vi "4155C Transfer Config SMUs.vi"(0 "VISA resource name in":refnum<visa-resource-name>, 1 "sweep method":u16(ring) items=["Continuous", "Pulsed"], 2 "Gate mode":u16(ring) items=["Auto", "Limited", "Fixed"], 3 "Gate Range":u8(slide)=6 max=11 scale=0.0..11.0, 5 "Pulse period":dbl=0.005 min=0.005 max=1.0 step=0.0001 format="%.4f", 7 "Pulse width":dbl=0.0005 min=0.0005 max=0.1 step=0.0001 format="%.4f", 8 "Drain Standby":bool, 9 "Base voltage":dbl format="%^.4e", 10 "Gate Standby":bool, 11 "error in (no error)":errorcluster, 12 "SMU4":cluster{"on/off":bool, "Voltage":dbl} {"Voltage" min=-100.0 max=100.0 format="%.2f"}, 13 "Source/drain mode":u16(ring) items=["Auto", "Limited", "Fixed"], 14 "Source/drain Range":u8(slide)=6 max=11 scale=0.0..11.0) -> (4 "VISA Resource Name out":refnum<visa-resource-name>, 15 "error out":errorcluster)   [LabVIEW 2016]
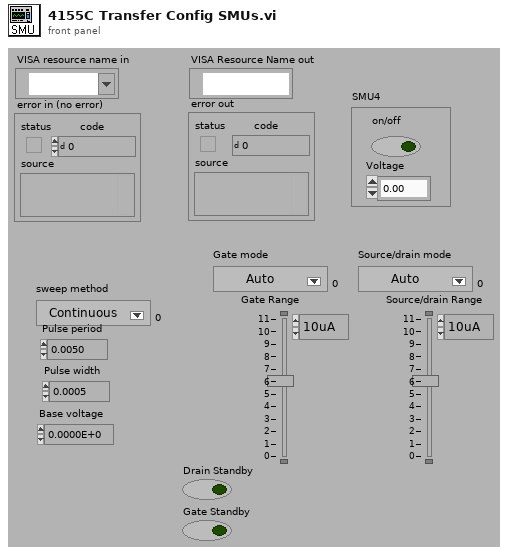
[diagram p1: front panel]
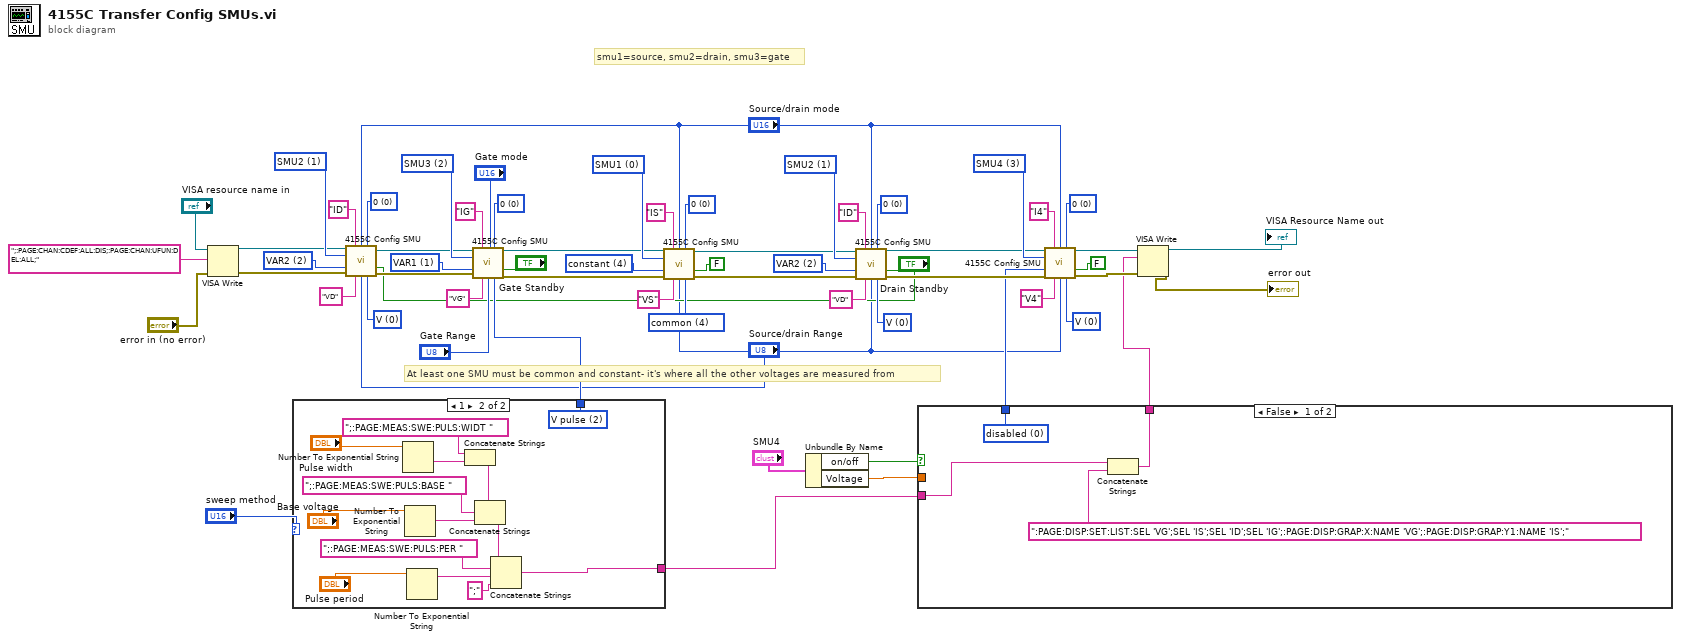
[diagram p0: block diagram]
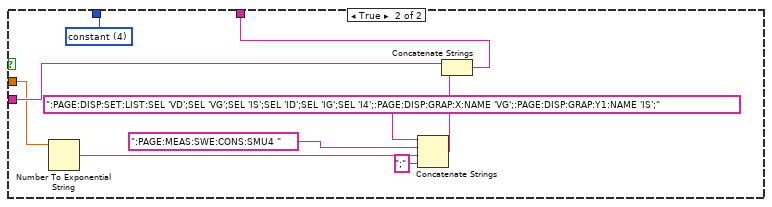
[diagram p2: hidden frame]
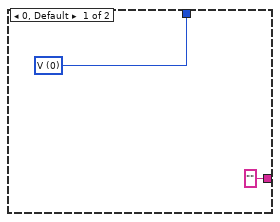
[diagram p3: hidden frame]
diagram:
  w18 = u32 1 items=["SMU1  ", "SMU2  ", "SMU3  ", "SMU4  ", "SMU5  ", "SMU6  "] ("unit to configure")
  w19 = u32 2 items=["disabled  ", "VAR1  ", "VAR2  ", "VAR1'  ", "constant  "] ("function")
  w21 = u32 0 items=["0  ", "10K Ohms  ", "100K Ohms  ", "1M Ohms  "] ("series resistance *")
  w22 = u32 0 items=["V  ", "I  ", "V pulse  ", "I pulse  ", "  common  "] ("mode")
  w40 = u32 0 items=["V  ", "I  ", "V pulse  ", "I pulse  ", "  common  "] ("mode")
  w41 = u32 0 items=["0  ", "10K Ohms  ", "100K Ohms  ", "1M Ohms  "] ("series resistance *")
  w43 = u32 3 items=["SMU1  ", "SMU2  ", "SMU3  ", "SMU4  ", "SMU5  ", "SMU6  "] ("unit to configure")
  w46 = u32 0 items=["0  ", "10K Ohms  ", "100K Ohms  ", "1M Ohms  "] ("series resistance *")
  w15 = u32 1 items=["disabled  ", "VAR1  ", "VAR2  ", "VAR1'  ", "constant  "] ("function")
  w48 = u32 2 items=["SMU1  ", "SMU2  ", "SMU3  ", "SMU4  ", "SMU5  ", "SMU6  "] ("unit to configure")
  w50 = u32 0 items=["V  ", "I  ", "V pulse  ", "I pulse  ", "  common  "] ("mode")
  w51 = u32 0 items=["0  ", "10K Ohms  ", "100K Ohms  ", "1M Ohms  "] ("series resistance *")
  w53 = u32 2 items=["disabled  ", "VAR1  ", "VAR2  ", "VAR1'  ", "constant  "] ("function")
  w54 = u32 1 items=["SMU1  ", "SMU2  ", "SMU3  ", "SMU4  ", "SMU5  ", "SMU6  "] ("unit to configure")
  w57 = u32 4 items=["V  ", "I  ", "V pulse  ", "I pulse  ", "  common  "] ("mode")
  w58 = u32 0 items=["0  ", "10K Ohms  ", "100K Ohms  ", "1M Ohms  "] ("series resistance *")
  w60 = u32 4 items=["disabled  ", "VAR1  ", "VAR2  ", "VAR1'  ", "constant  "] ("function")
  w61 = u32 0 items=["SMU1  ", "SMU2  ", "SMU3  ", "SMU4  ", "SMU5  ", "SMU6  "] ("unit to configure")
  # "smu1=source, smu2=drain, smu3=gate"
  # "At least one SMU must be common and constant- it's where all the other voltages are measured from"
  n1 = VISA Write(VISA resource name="VISA resource name in", write buffer=";:PAGE:CHAN:CDEF:ALL:DIS;:PAGE:CHAN:UFUN:DEL:ALL;", error in (no error)="error in (no error)") -> (VISA resource name out=w3:refnum<visa-resource-name>, error out=w1:errorcluster)  [unwired: 1 out]
  n2 = case shown="1" "sweep method" {
    tunnel: [w63 w77] -> w30
    tunnel: ["" w65] -> w14
    frame 0, Default {
      w63 = u32 0 items=["V  ", "I  ", "V pulse  ", "I pulse  ", "  common  "] ("mode")
    }
    frame 1 {
      w77 = u32 2 items=["V  ", "I  ", "V pulse  ", "I pulse  ", "  common  "] ("mode")
      n3 = Number To Exponential String(number="Pulse width") -> (E-format string=w73:string)  [unwired: 3 in]
      n4 = Number To Exponential String(number="Base voltage") -> (E-format string=w69:string)  [unwired: 3 in]
      n5 = Number To Exponential String(number="Pulse period") -> (E-format string=w66:string)  [unwired: 3 in]
      n6 = Concatenate Strings(";:PAGE:MEAS:SWE:PULS:WIDT " ("Substring"), w73) -> (w71:string)
      n7 = Concatenate Strings(w71, ";:PAGE:MEAS:SWE:PULS:BASE " ("Substring"), w69) -> (w67:string)
      n8 = Concatenate Strings(w67, ";:PAGE:MEAS:SWE:PULS:PER " ("Substring"), w66, ";" ("Substring")) -> (w65:string)
    }
  }
  n9 = call "4155C Config SMU.vi"("VISA session"=w3, "I name (max 6 chars)"="ID", "Range mode"="Source/drain mode", "series resistance *"=w21, "unit to configure"=w18, "function"=w19, "standby"="Drain Standby", "error in (no error)"=w1, "V name (max 6 chars)"="VD", "Range"="Source/drain Range", "mode"=w22) -> ("dup VISA resource name"=w16:refnum<visa-resource-name>, "error out"=w17:errorcluster)  [unwired: 3 in]
  n10 = call "4155C Config SMU.vi"("VISA session"=w16, "I name (max 6 chars)"="IG", "Range mode"="Gate mode", "series resistance *"=w46, "unit to configure"=w48, "function"=w15, "standby"="Gate Standby", "error in (no error)"=w17, "V name (max 6 chars)"="VG", "Range"="Gate Range", "mode"=w30) -> ("dup VISA resource name"=w27:refnum<visa-resource-name>, "error out"=w26:errorcluster)  [unwired: 3 in]
  n11 = call "4155C Config SMU.vi"("VISA session"=w27, "I name (max 6 chars)"="IS", "Range mode"="Source/drain mode", "series resistance *"=w58, "unit to configure"=w61, "function"=w60, "standby"=FALSE, "error in (no error)"=w26, "V name (max 6 chars)"="VS", "Range"="Source/drain Range", "mode"=w57) -> ("dup VISA resource name"=w37:refnum<visa-resource-name>, "error out"=w36:errorcluster)  [unwired: 3 in]
  n12 = Unbundle By Name("SMU4") -> ("on/off"=w12:bool, "Voltage"=w13:dbl)
  n13 = call "4155C Config SMU.vi"("VISA session"=w37, "I name (max 6 chars)"="ID", "Range mode"="Source/drain mode", "series resistance *"=w51, "unit to configure"=w54, "function"=w53, "standby"="Drain Standby", "error in (no error)"=w36, "V name (max 6 chars)"="VD", "Range"="Source/drain Range", "mode"=w50) -> ("dup VISA resource name"=w24:refnum<visa-resource-name>, "error out"=w25:errorcluster)  [unwired: 3 in]
  n14 = case shown="False" w12 {
    tunnel: w14 -> [w80 w90]
    tunnel: [w79 w89] -> w10
    tunnel: w13 -> [_ w87]
    tunnel: [w78 w88] -> w9
    frame False {
      w78 = u32 0 items=["disabled  ", "VAR1  ", "VAR2  ", "VAR1'  ", "constant  "] ("function")
      n15 = Concatenate Strings(w80, ":PAGE:DISP:SET:LIST:SEL 'VG';SEL 'IS';SEL 'ID';SEL 'IG';:PAGE:DISP:GRAP:X:NAME 'VG';:PAGE:DISP:GRAP:Y1:NAME 'IS';" ("write buffer (\"\")")) -> (w79:string)
    }
    frame True {
      w88 = u32 4 items=["disabled  ", "VAR1  ", "VAR2  ", "VAR1'  ", "constant  "] ("function")
      n16 = Number To Exponential String(number=w87) -> (E-format string=w85:string)  [unwired: 3 in]
      n17 = Concatenate Strings(":PAGE:DISP:SET:LIST:SEL 'VD';SEL 'VG';SEL 'IS';SEL 'ID';SEL 'IG';SEL 'I4';:PAGE:DISP:GRAP:X:NAME 'VG';:PAGE:DISP:GRAP:Y1:NAME 'IS';" ("write buffer (\"\")"), ":PAGE:MEAS:SWE:CONS:SMU4 " ("write buffer (\"\")"), w85, ";" ("Substring")) -> (w83:string)
      n18 = Concatenate Strings(w90, w83) -> (w89:string)
    }
  }
  n19 = call "4155C Config SMU.vi"("VISA session"=w24, "I name (max 6 chars)"="I4", "Range mode"="Source/drain mode", "series resistance *"=w41, "unit to configure"=w43, "function"=w9, "standby"=FALSE, "error in (no error)"=w25, "V name (max 6 chars)"="V4", "Range"="Source/drain Range", "mode"=w40) -> ("dup VISA resource name"=w35:refnum<visa-resource-name>, "error out"=w34:errorcluster)  [unwired: 3 in]
  n20 = VISA Write(VISA resource name=w35, write buffer=w10, error in (no error)=w34) -> (VISA resource name out=→"VISA Resource Name out":refnum<visa-resource-name>, error out=→"error out":errorcluster)  [unwired: 1 out]
